vi "New Client.vi"(8 "error in (no error)":errorcluster, 10 "Port":u16, 11 "Communication Clients in":refnum<class "Communication Clients.lvclass">) -> (0 "error out":errorcluster, 3 "Communication Clients out":refnum<class "Communication Clients.lvclass">)   [LabVIEW 2017, in "Communication Clients.lvlib" / "Communication Clients.lvclass"]
uses:
  Communication Clients.lvclass
  C:/Program Files (x86)/National Instruments/LabVIEW 2017/vi.lib/ActorFramework/Actor/Actor.lvclass
  Communication Clients Messages/New Message Msg/New Message Msg.lvclass
  C:/Users/Public/Documents/wc/BuildFarm/src/LabVIEW/vi.lib/BenjaminR/Build Farm/Actors/Communication/WebSocket Client/WebSocket Client Messages/New Message Msg/New Message Msg.lvclass
  src/LabVIEW/vi.lib/BenjaminR/Build Farm/Actors/Communication/WebSocket Client/WebSocket Client/WebSocket Client.lvclass/WebSocket Client.ctl
  Communication Clients.lvclass/Communication Clients.ctl
  src/LabVIEW/vi.lib/BenjaminR/Build Farm/Actors/Communication/WebSocket Client/WebSocket Client/WebSocket Client.lvclass
  <vilib>/ActorFramework/Actor/Actor.lvclass
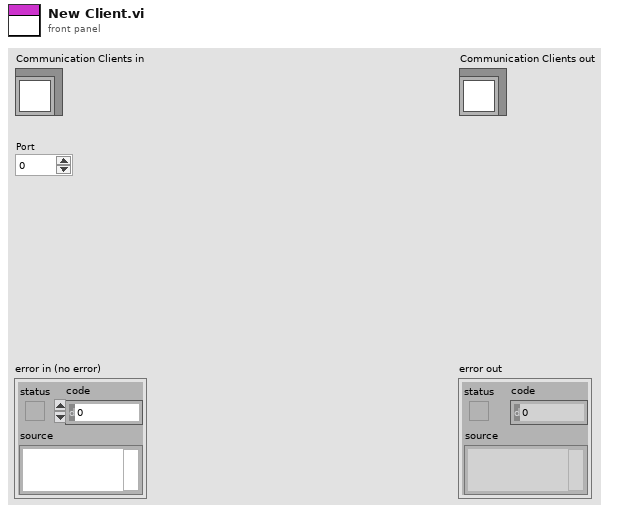
[diagram p1: front panel]
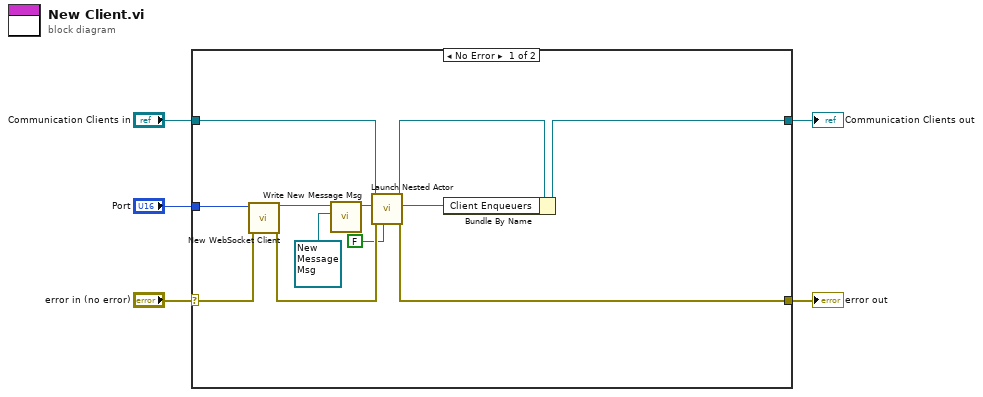
[diagram p0: block diagram]
diagram:
  n1 = case shown="No Error" "error in (no error)" {
    selector: "error in (no error)" -> [w8 w19]
    tunnel: [w9 w19] -> w4
    tunnel: [w12 w18] -> w2
    tunnel: "Communication Clients in" -> [w14 w18]
    tunnel: "Port" -> [w17 _]
    frame No Error {
      n2 = call "New WebSocket Client.vi"("error in (no error)"=w8, "Port"=w17) -> ("error out"=w10:errorcluster, "WebSocket Client out"=w16:refnum<class "WebSocket Client.lvclass">)  [unwired: 8 in]
      n3 = call "Write New Message Msg.vi"("WebSocket Client.lvlib:New Message Msg.lvclass"=refnum<class "New Message Msg.lvclass"> refnum ("Communication Clients.lvlib:New Message Msg.lvclass"), "WebSocket Client in"=w16) -> ("WebSocket Client out"=w13:refnum<class "WebSocket Client.lvclass">)  [unwired: 9 in]
      n4 = call <vilib>:"Launch Nested Actor.vi"("Open Actor Core front panel? (F)"=FALSE, "error in (no error)"=w10, "Nested Actor"=w13, "Caller Actor in"=w14) -> ("error out"=w9:errorcluster, "Nested Actor's Enqueuer"=w6:refnum<class "Message Enqueuer.lvclass">, "Caller Actor out"=w11:refnum<class "Communication Clients.lvclass">)  [unwired: 5 in]
      n5 = Bundle By Name(cluster=w11, "Client Enqueuers"=w6) -> (w12:refnum<class "Communication Clients.lvclass">)
    }
    frame Error {
    }
  }
  "error out" <- w4
  "Communication Clients out" <- w2
